vi "ABB Test Heat run.vi"(10 "Measure":enum16{"Full Load", "Partial Load", "No Load"}(ring), 11 "Heat run Type":enum16{"Full Load", "Partial- & No-Load"}(ring)) -> ()   [LabVIEW 2017]
uses:
  Temp error msg.ctl
  Video Display Buttons.ctl
  <vilib>/Analysis/baseanly.llb/Mean (DBL).vi
  ABB global.vi
  <vilib>/Analysis/NI_AALBase.lvlib
panel:
  in  "Video Displays":T1
  in  "Temp error":T2="Error: Temperature measurement "
  out "Additional Temperatures 2":string[][](table)
  out "Bearing Run readings":string[][](table)
  in  "Rated":T3
  in  "copying":string="Copying.."
  in  "copy to bearing":bool
  in  "Averaging":i32=1 min=1 max=1000
  in  "Smooth power\n    readings":bool
  in  "Reading Category":T4(ring)=enum."Wdg Temp"
  out "Power Readings":string[][](table)
  in  "Comments":string
  in  "Start":bool
  out "Type of Run":string
  out "Additional Temperatures":string[][](table)
  in  "Stabilitymessg":string="Thermal Stability reached"
  out "Time to Next reading":dbl(slide) scale=0.0..30.0 scale format="%#.1f"
  out "Start Time":dbl
  out "Temperatures":string[][](table)
  out "Readings":string[][](table)
  out "saved Readings":dbl[][](array[numeric])
  out "Serial number":string
  out "W.O number":string
  out "Norma 5000 Error":string
  in  "Record":bool
  out "Readings Table":string[][](table)
  in  "View":enum16{"Graph", "Readings"}(ring)
  out "Number readings":i32
  out "Status":enum16{"Stopped", "Running", "Finished"}(ring)
  out "Timedate":string
  in  "End test":bool
  in  "Read Mode":enum16{"Auto", "Manual"}(ring)
  in  "Exit":bool
  out "Temperature Trend":cluster{dbl[], "Best Linear Fit":dbl[]}[](graph)
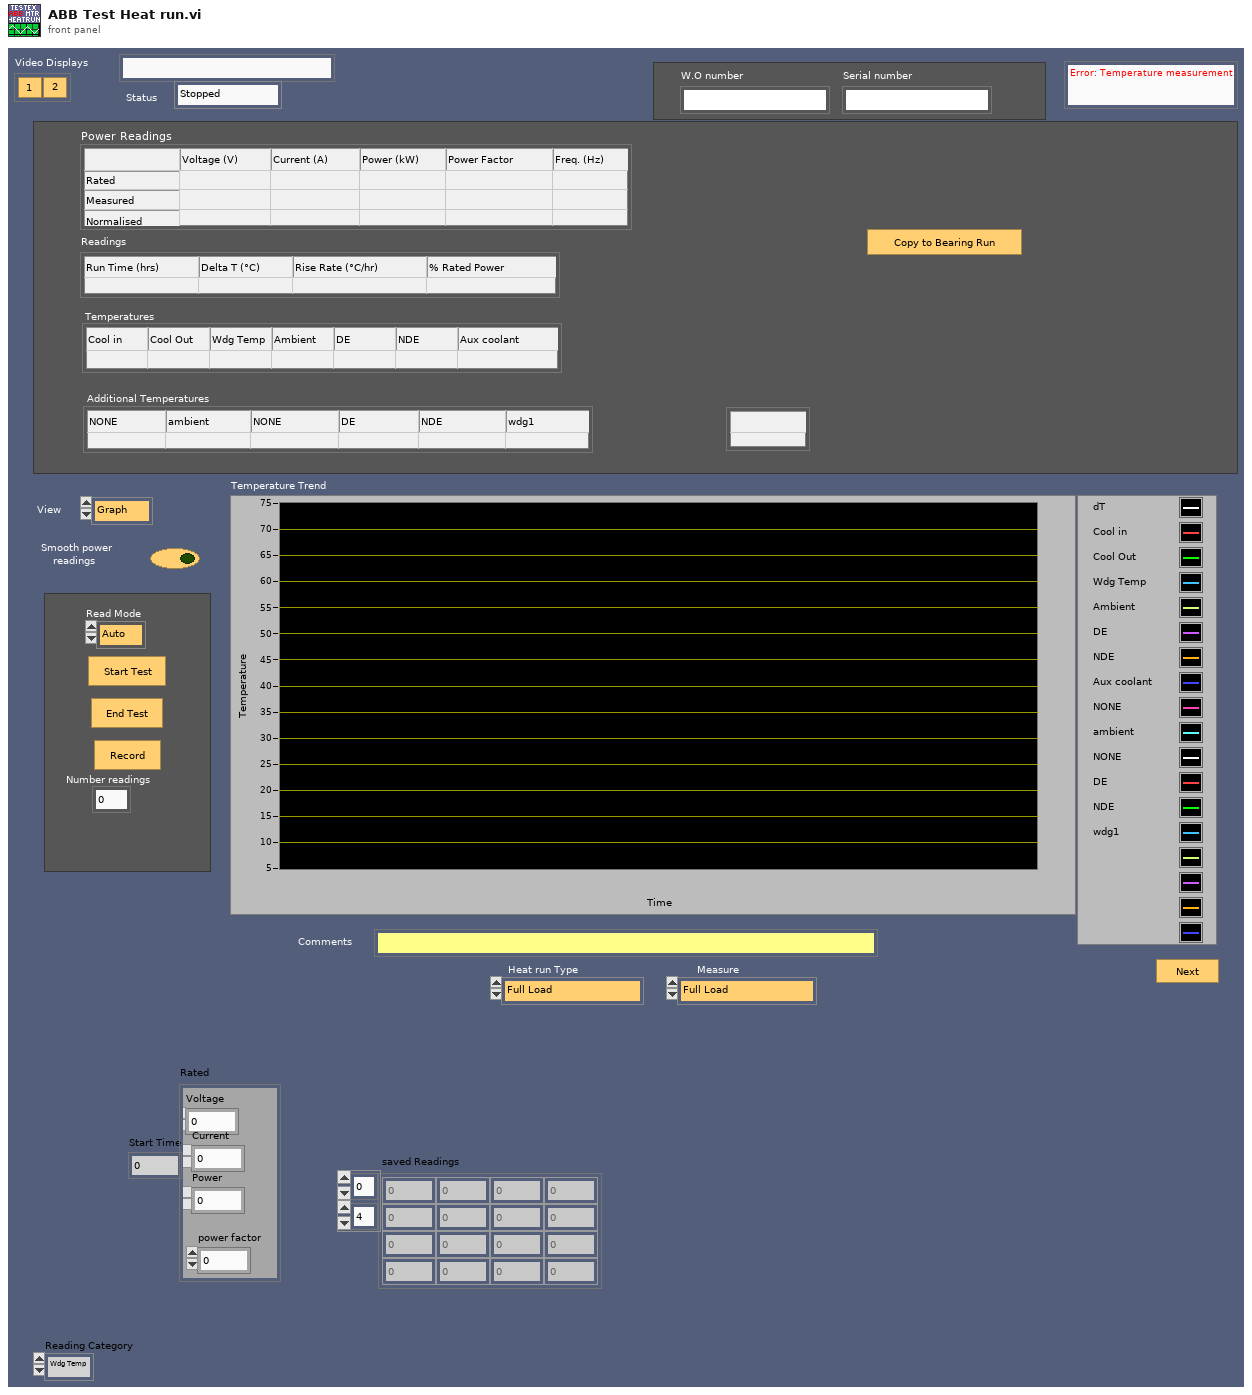
[diagram p1: front panel]
types:
  T1 = typedef "Video Display Buttons.ctl" = cluster{"1":bool, "1 2":bool}
  T2 = typedef "Temp error msg.ctl" = string
  T3 = cluster{"Voltage":dbl, "Current":dbl, "Power":dbl, "power factor":dbl}
  T4 = enum16{"None", "Cool in", "Cool Out", "Wdg Temp", "Ambient", "DE", "NDE", "Aux coolant"}
  T5 = enum16{"No load", "Locked Rotor", "Heat run", "NoLd heat run", "Partial heat run"}
  T6 = enum16{"Heat run", "Bearing run", "NoLd Heat Run", "Partial heat run"}
  T7 = cluster{"VT Primary":dbl, "VT Secondary":dbl, "CT  Primary":dbl, "CT Secondary":dbl, "Current Shunt":enum16{"Internal", "External"}, "Avg interval":dbl}
  T8 = cluster{"VT Primary":dbl, "VT Secondary":dbl, "CT  Primary":dbl, "CT Secondary":dbl, "Current Shunt":enum16{"Internal", "External"}, "Averaging interval (secs)":dbl}
  T9 = cluster{"Visa sesssion":refnum<visa-resource-name>, "error":errorcluster}
  T10 = cluster{"Simulate Norma":bool, "Norma 5000 Address":u8, "WebDaq IP Address":string, "Simulate cDAQ":bool}
  T11 = cluster{"Thermal Stability (deg/hr)":dbl, "Reading interval (mins)":dbl}
  T12 = cluster{"String":string, "String":string, "String":string, "String":string}
  T13 = cluster{"String":dbl, "String":dbl, "String":dbl, "String":dbl}
  T14 = cluster{"temp. alloc":i32[], "category":i32[], "Category names":string[], "Category none names":string[]}
  T15 = cluster{"V":dbl, "A":dbl, "W":dbl, "VA":dbl, "VAr":dbl, "Pf":dbl}
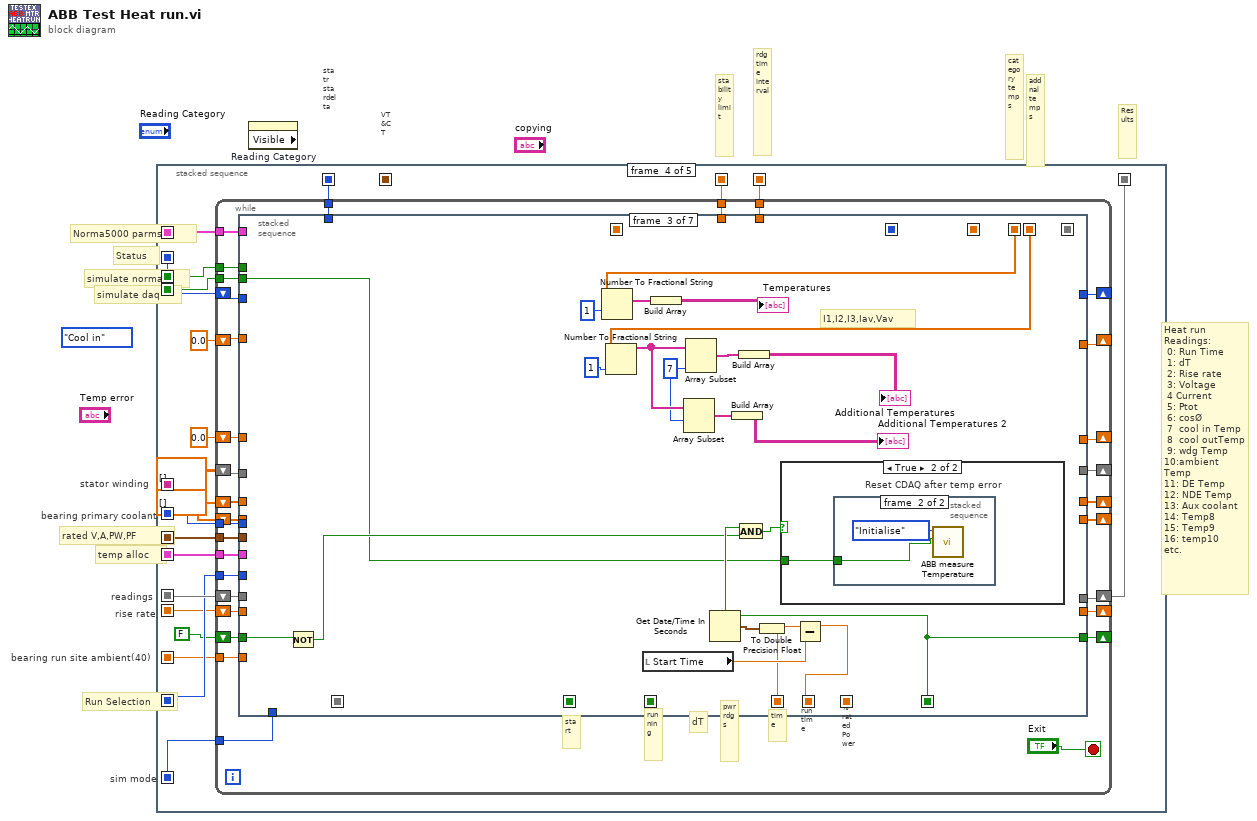
[diagram p0: block diagram]
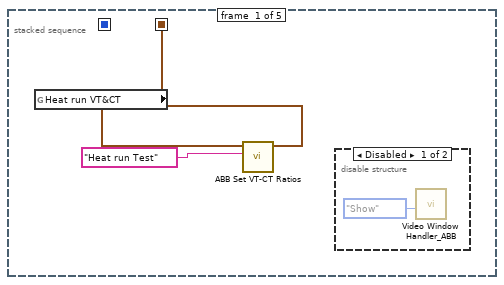
[diagram p2: hidden frame]
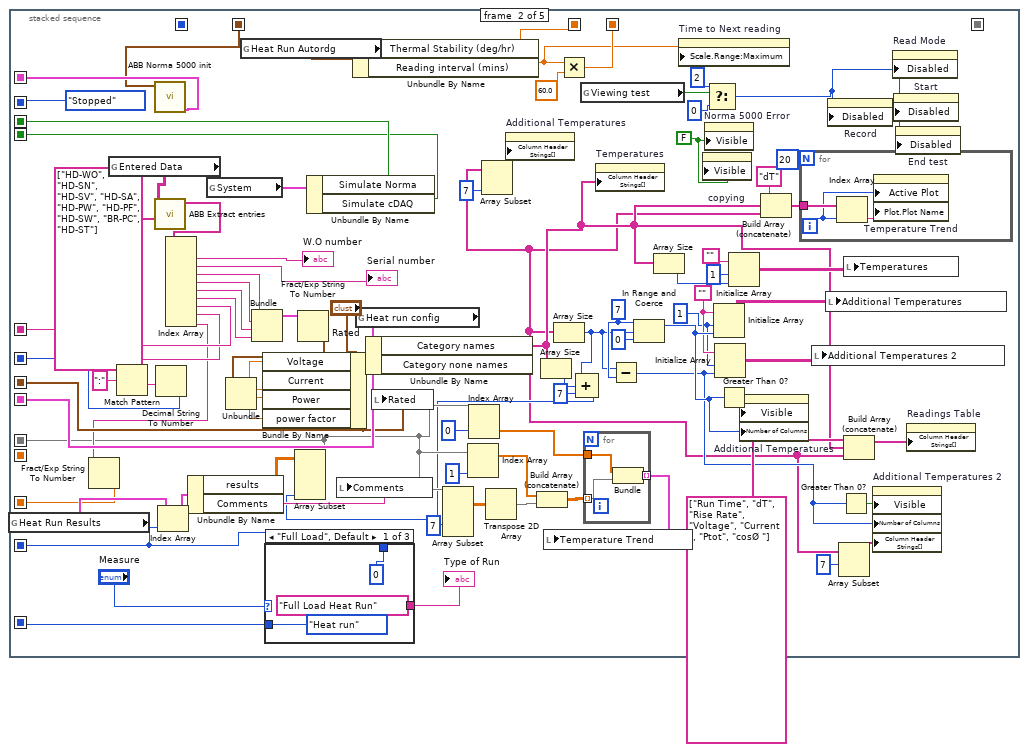
[diagram p4: hidden frame]
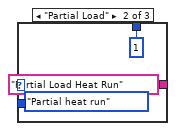
[diagram p5: hidden frame]
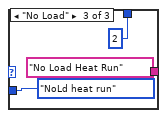
[diagram p6: hidden frame]
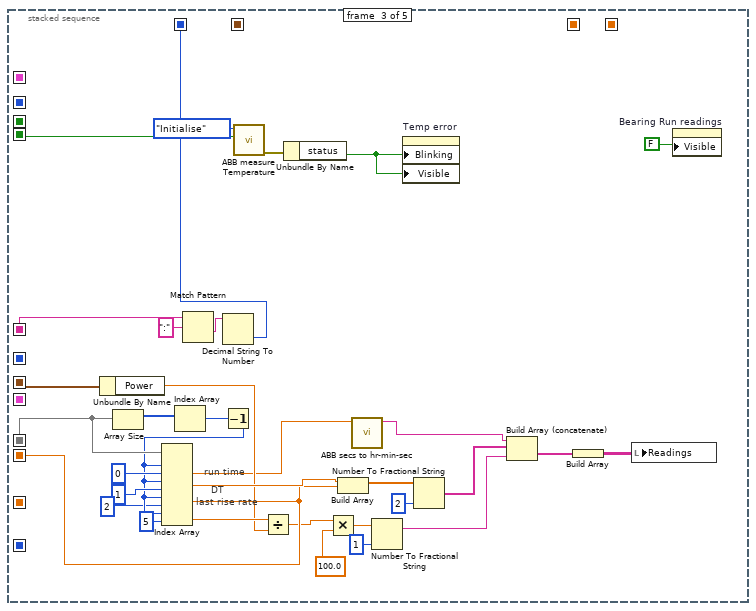
[diagram p7: hidden frame]
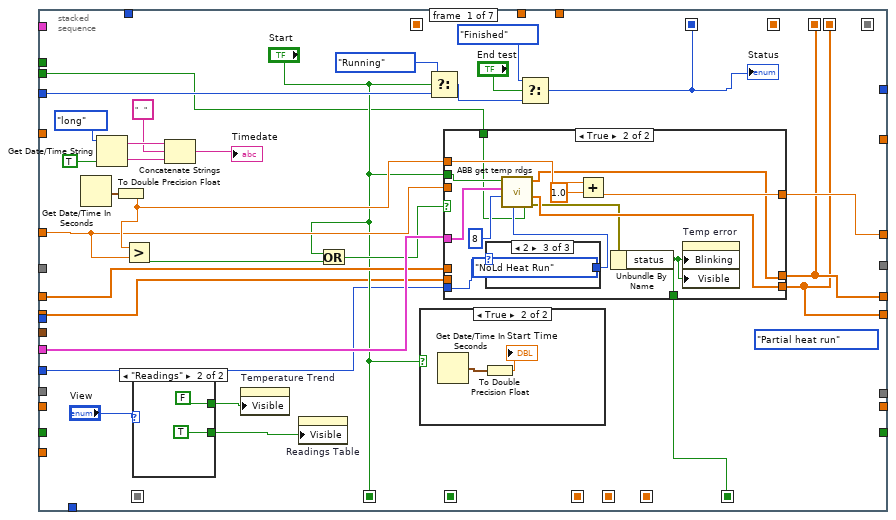
[diagram p8: hidden frame]
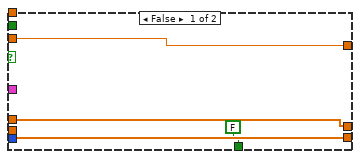
[diagram p10: hidden frame]
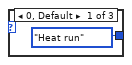
[diagram p11: hidden frame]
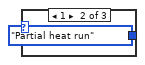
[diagram p12: hidden frame]
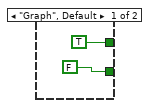
[diagram p13: hidden frame]
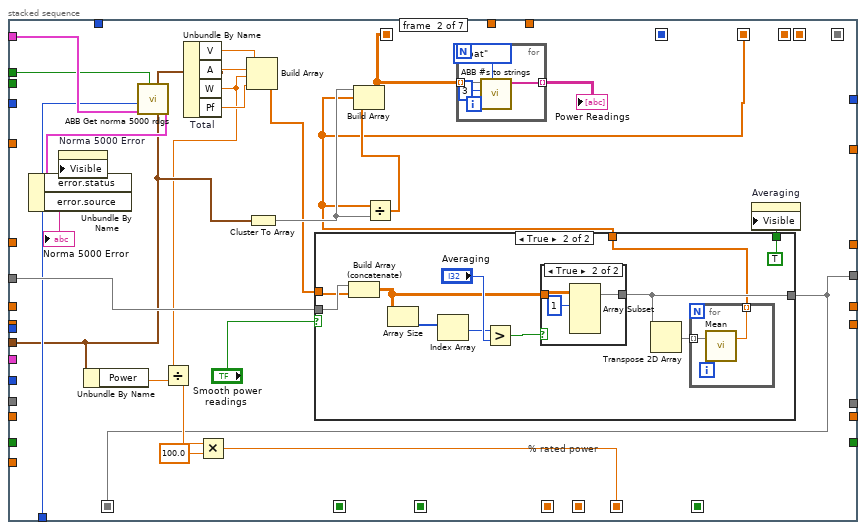
[diagram p14: hidden frame]
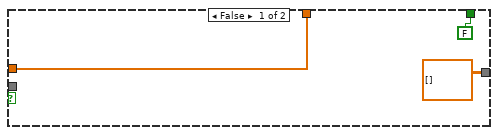
[diagram p15: hidden frame]
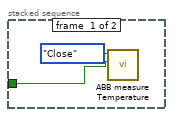
[diagram p18: hidden frame]
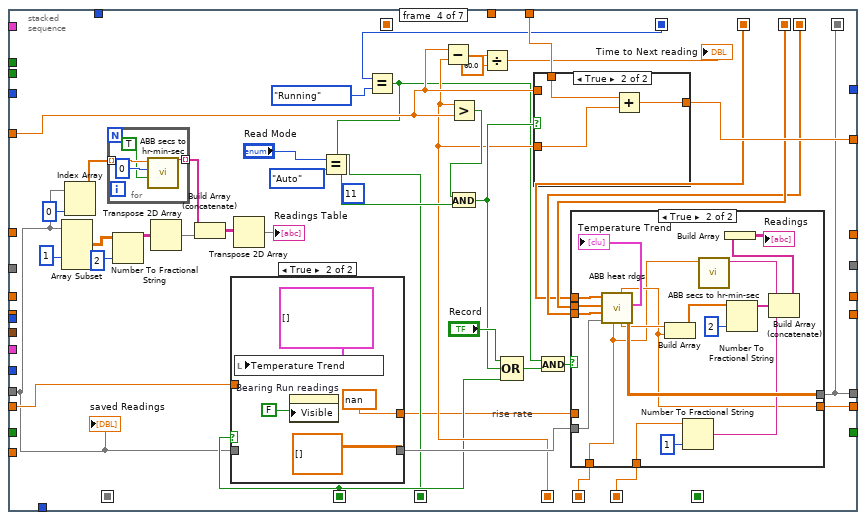
[diagram p19: hidden frame]
diagram:
  (unwired) T4."Cool in" ("Reading Category")
  # "bearing run site ambient(40)"
  # "bearing primary coolant"
  # "VT&CT"
  # "statr stardelta"
  # "stator winding"
  # "rise rate"
  # "readings"
  # "sim mode"
  # "simulate daq"
  # "addnal temps"
  # "category temps"
  # "Run Selection"
  # "stability limit"
  # "Results"
  # "rdg time interval"
  # "Heat run Readings:\n 0: Run Time\n 1: dT\n 2: Rise rate\n 3: Voltage\n 4 Current\n 5: Ptot\n 6: cosØ\n 7  cool in Temp\n 8  cool outTemp\n 9: wdg Temp\n10:ambient Temp\n11: DE Temp\n12: NDE Temp\n13: Aux coolant\n14: Temp8\n15: Temp9\n16: temp10\netc."
  # "temp alloc"
  # "rated V,A,PW,PF"
  # "simulate norma"
  # "Norma5000 parms"
  # "Status"
  n1 = stacked-sequence {
    seq-local: [_ enum16{"Stopped", "Running", "Finished"}."Stopped" ("Status") _ _ _] -> [_ _ _ w162 _]
    seq-local: [_ w91 _ _ _] -> [_ _ _ w161 w476]
    seq-local: [_ w89 _ _ _] -> [_ _ _ w160 w475]
    seq-local: [_ w39 _ _ _] -> [_ _ w130 w159 _]
    seq-local: [_ w8 _ _ _] -> [_ _ w139 w158 _]
    seq-local: [_ w54 _ _ _] -> [_ _ _ w156 _]
    seq-local: [_ w76 _ _ _] -> [_ _ _ w155 _]
    seq-local: [_ _ _ w153 _] -> [_ _ _ _ w473]
    seq-local: [_ w66 _ _ _] -> [_ _ _ w152 _]
    seq-local: [_ w48 _ _ _] -> [_ _ _ w149 w472]
    seq-local: [_ w52 _ _ _] -> [_ _ w111 w147 w469]
    seq-local: [_ w46 _ _ _] -> [_ _ _ w148 _]
    seq-local: [_ _ w133 _ _] -> [_ _ _ w146 _]
    seq-local: [_ w31 _ _ _] -> [_ _ w114 _ _]
    seq-local: [_ _ w113 _ _] -> [_ _ _ w145 _]
    seq-local: [w2 _ _ _ _] -> [_ w32 _ _ w471]
    seq-local: [_ w27 _ _ _] -> [_ _ _ w144 _]
    seq-local: [_ w25 _ _ _] -> [_ _ _ w143 _]
    frame #0 {
      n2 = global read "ABB global.vi" "Heat run VT&CT"() -> (w3:T7)
      n3 = call "ABB Set VT-CT Ratios.vi"("Test name"="Heat run Test", "VT and CT Ratios"=w3) -> ("VT and CT Ratios out"=w2:T8)  [unwired: 9 in]
      n4 = disable-structure shown="Disabled" {
        frame Disabled {
          n5 = call "Video Window Handler_ABB.vi"("Action"=enum16{"Show", "Hide", "Exit"}."Show") -> ()  [unwired: 11 in]
        }
        frame Enabled {
        }
      }
    }
    frame #1 {
      w22 = 7 ("upper limit")
      w21 = ""
      w20 = 1 ("dimension size")
      w53 = FALSE ("Visible")
      n6 = global read "ABB global.vi" "Heat Run Results"() -> (w49:cluster{"results":dbl[][], "Comments":string}[])
      n7 = global read "ABB global.vi" "Entered Data"() -> (w72:string[][])
      n8 = call "ABB Norma 5000 init.vi"("VT and CT Ratios"=w32) -> ("norma 5000 parms out"=w91:T9)  [unwired: 10 in]
      n9 = call "ABB Extract entries.vi"("Entry IDs"=string[] ["HD-WO", "HD-SN", "HD-SV", "HD-SA", "HD-PW", "HD-PF", "HD-SW", "BR-PC", "HD-ST"], "Entry table in"=w72) -> ("Selected Entries"=w38:string[])  [unwired: 9 in]
      n10 = Index Array(array=w38) -> (element #1=→"W.O number":string, element #2=→"Serial number":string, element #3=w68:string, element #4=w56:string, element #5=w55:string, element #6=w57:string, element #7=w31:string, element #8=w28:string, element #9=w26:string)  [unwired: 9 in]
      n11 = Fract/Exp String To Number(string=w26) -> (number=w25:dbl)  [unwired: 3 in, 1 out]
      n12 = Match Pattern(string=w28, regular expression=":") -> (after substring=w29:string)  [unwired: 1 in, 3 out]
      n13 = Decimal String To Number(string=w29) -> (number=w27:i32)  [unwired: 2 in, 1 out]
      n14 = global read "ABB global.vi" "System"() -> (w90:T10)
      n15 = global read "ABB global.vi" "Heat Run Autordg"() -> (w88:T11)
      n16 = Bundle("String"=w68, "String"=w56, "String"=w55, "String"=w57) -> (w67:T12)  [unwired: 1 in]
      n17 = case shown="\"Full Load\", Default" "Measure" {
        tunnel: ["Full Load Heat Run" "Partial Load Heat Run" "No Load Heat Run"] -> w51
        tunnel: [0 1 2] -> w48
        tunnel: [T5."Heat run" ("Simulate Mode") T5."Partial heat run" ("Simulate Mode") T5."NoLd heat run" ("Simulate Mode")] -> w46
        frame "Full Load", Default {
        }
        frame "Partial Load" {
        }
        frame "No Load" {
        }
      }
      "Type of Run" <- w51
      n18 = Index Array(array=w49, index=w48) -> (element=w62:cluster{"results":dbl[][], "Comments":string})
      n19 = Unbundle By Name(w62) -> ("results"=w9:dbl[][], "Comments"=w50:string)
      n20 = Fract/Exp String To Number(string=w67) -> (number=w44:T13)  [unwired: 3 in, 1 out]
      n21 = Unbundle(w44) -> ("String"=w43:dbl, "String"=w42:dbl, "String"=w41:dbl, "String"=w40:dbl)
      n22 = Bundle By Name(cluster="Rated", "Voltage"=w43, "Current"=w42, "Power"=w41, "power factor"=w40) -> (w39:T3)
      n23 = Unbundle By Name(w90) -> ("Simulate Norma"=w89:bool, "Simulate cDAQ"=w52:bool)
      n24 = local write "Comments"(w50) -> ()
      n25 = Unbundle By Name(w88) -> ("Thermal Stability (deg/hr)"=w66:dbl, "Reading interval (mins)"=w75:dbl)
      n26 = global read "ABB global.vi" "Heat run config"() -> (w54:T14)
      n27 = Unbundle By Name(w54) -> ("Category names"=w6:string[], "Category none names"=w5:string[])
      n28 = local write "Rated"(w39) -> ()
      n29 = Array Subset(array=w5, length=7) -> (w16:string[])  [unwired: 1 in]
      n30 = property on="Additional Temperatures" class="Tbl (strict)"("Column Header Strings[]"=w16) -> ()  [unwired: 2 in, 2 out]
      n31 = Array Size(array=w6) -> (size(s)=w12:i32)
      n32 = Array Size(array=w5) -> (size(s)=w11:i32)
      n33 = Multiply(x=w75, y=60.0) -> (x*y=w76:dbl)
      n34 = Compound Arithmetic op=ADD(w11, w12, 7 ("value")) -> (w7:i32)
      n35 = Array Subset(array=w9, length (col)=w7) -> (w8:dbl[][])  [unwired: 3 in]
      n36 = Array Subset(array=w8, index (col)=7 ("index")) -> (w79:dbl[][])  [unwired: 3 in]
      n37 = Index Array(array=w8, index (col)=1 ("disabled index (col)")) -> (element=w33:dbl[])  [unwired: 1 in]
      n38 = Index Array(array=w8, index (col)=0 ("disabled index (col)")) -> (element=w81:dbl[])  [unwired: 1 in]
      n39 = Transpose 2D Array(2D array=w79) -> (transposed array=w78:dbl[][])
      n40 = Build Array (concatenate)(w33, w78) -> (w34:dbl[][])
      n41 = global read "ABB global.vi" "Viewing test"() -> (w61:bool)
      n42 = for {
        tunnel: w81 -> [w104]
        tunnel: w34 -> [w103] mode=indexing
        tunnel: [w102] -> w77 mode=indexing
        n43 = Bundle(w104, w103) -> (w102:cluster{dbl[], dbl[]})  [unwired: 1 in]
      }
      n44 = local write "Temperature Trend"(w77) -> ()
      n45 = property on="Temperatures" class="Tbl (strict)"("Column Header Strings[]"=w6) -> ()  [unwired: 2 in, 2 out]
      n46 = Subtract(x=w11, y=w22) -> (x-y=w17:i32)
      n47 = In Range and Coerce(upper limit=w22, x=w11, lower limit=0) -> (coerced(x)=w24:i32)  [unwired: 1 out]
      n48 = Array Size(array=w6) -> (size(s)=w86:i32)
      n49 = property on="Time to Next reading" class="Slide (strict)"("Scale.Range:Maximum"=w75) -> ()  [unwired: 2 in, 2 out]
      n50 = property on="copying" class="Str"("Visible"=w53) -> ()  [unwired: 2 in, 2 out]
      n51 = property on="Norma 5000 Error" class="Str"("Visible"=w53) -> ()  [unwired: 2 in, 2 out]
      n52 = Select(t=2, s=w61, f=0) -> (s? t:f=w58:i32)
      n53 = Initialize Array(w21, w20, w24) -> (w65:string[][])
      n54 = Initialize Array(w21, w20, w17) -> (w19:string[][])
      n55 = Greater Than 0?(x=w24) -> (x > 0?=w64:bool)
      n56 = Initialize Array("", 1 ("dimension size"), w86) -> (w84:string[][])
      n57 = property on="Additional Temperatures" class="Tbl (strict)"("Visible"=w64, "Number of Columns"=w24) -> ()  [unwired: 2 in, 2 out]
      n58 = Build Array (concatenate)("dT", w6, w5) -> (w37:string[])
      n59 = for {
        N: 20 -> [_]
        tunnel: w37 -> [w107]
        i -> [w106]
        n60 = Index Array(array=w107, index=w106) -> (element=w105:string)
        n61 = property on="Temperature Trend" class="XYGraph (strict)"("Active Plot"=w106, "Plot.Plot Name"=w105) -> ()  [unwired: 2 in, 2 out]
      }
      n62 = local write "Additional Temperatures 2"(w19) -> ()
      n63 = local write "Additional Temperatures"(w65) -> ()
      n64 = property on="Record" class="Bool"("Disabled"=w58) -> ()  [unwired: 2 in, 2 out]
      n65 = Array Subset(array=w5, index=7) -> (w13:string[])  [unwired: 1 in]
      n66 = Greater Than 0?(x=w17) -> (x > 0?=w18:bool)
      n67 = local write "Temperatures"(w84) -> ()
      n68 = Build Array (concatenate)(string[] ["Run Time", "dT", "Rise Rate", "Voltage", "Current ", "Ptot", "cosØ "], w6, w5) -> (w73:string[])
      n69 = property on="Additional Temperatures 2" class="Tbl (strict)"("Visible"=w18, "Number of Columns"=w17, "Column Header Strings[]"=w13) -> ()  [unwired: 2 in, 2 out]
      n70 = property on="Read Mode" class="Enum (strict)"("Disabled"=w58) -> ()  [unwired: 2 in, 2 out]
      n71 = property on="Start" class="Bool"("Disabled"=w58) -> ()  [unwired: 2 in, 2 out]
      n72 = property on="End test" class="Bool"("Disabled"=w58) -> ()  [unwired: 2 in, 2 out]
      n73 = property on="Readings Table" class="Tbl (strict)"("Column Header Strings[]"=w73) -> ()  [unwired: 2 in, 2 out]
    }
    frame #2 {
      # "DT"
      # "run time"
      # "last rise rate"
      n74 = Unbundle By Name(w130) -> ("Power"=w129:dbl)
      n75 = Array Size(array=w139) -> (size(s)=w141:i32[])
      n76 = Index Array(array=w141) -> (element=w140:i32)  [unwired: 1 in]
      n77 = Match Pattern(string=w114, regular expression=":") -> (after substring=w115:string)  [unwired: 1 in, 3 out]
      n78 = Decimal String To Number(string=w115) -> (number=w113:i32)  [unwired: 2 in, 1 out]
      n79 = Decrement(x=w140) -> (x-1=w136:i32)
      n80 = Index Array(array=w139, index (row) #1=w136, index (col) #1=0, index (row) #2=w136, index (col) #2=1 ("disabled index (col)"), index (row) #3=w136, index (col) #3=2 ("disabled index (col)"), index (row) #4=w136, index (col) #4=5 ("disabled index (col)")) -> (element #1=w118:dbl, element #2=w135:dbl, element #3=w133:dbl, element #4=w131:dbl)
      n81 = call "ABB measure Temperature.vi"("Simulate"=w111, "Mode"=enum16{"Initialise", "Read", "Close"}."Initialise") -> ("error out"=w109:errorcluster)  [unwired: 7 in, 2 out]
      n82 = Divide(x=w131, y=w129) -> (x/y=w126:dbl)
      n83 = Unbundle By Name(w109) -> ("status"=w108:bool)
      n84 = Multiply(x=w126, y=100.0) -> (x*y=w120:dbl)
      n85 = Build Array(w135, w133) -> (w128:dbl[])
      n86 = call "ABB secs to hr-min-sec.vi"("Seconds"=w118) -> ("hr:min:secs"=w117:string)  [unwired: 10 in]
      n87 = Number To Fractional String(number=w120, precision (6)=i16 1) -> (F-format string=w123:string)  [unwired: 2 in]
      n88 = property on="Temp error" class="Str (strict)"("Blinking"=w108, "Visible"=w108) -> ()  [unwired: 2 in, 2 out]
      n89 = Number To Fractional String(number=w128, precision (6)=i16 2) -> (F-format string=w124:string[])  [unwired: 2 in]
      n90 = Build Array (concatenate)(w117, w124, w123) -> (w122:string[])
      n91 = Build Array(w122) -> (w121:string[][])
      n92 = local write "Readings"(w121) -> ()
      n93 = property on="Bearing Run readings" class="Tbl (strict)"("Visible"=FALSE) -> ()  [unwired: 2 in, 2 out]
    }
    frame #3 {
      w151 = dbl[] []
      n94 = while {
        shift-right: [w191] -> _
        shift-left: w162 -> [w192]
        tunnel: w161 -> [w190]
        tunnel: w160 -> [w189]
        tunnel: w159 -> [w188]
        shift-right: [w186] -> w153
        shift-left: w158 -> [w187]
        shift-right: [w183] -> _
        shift-left: 0.0 -> [w185]
        shift-right: [w184] -> _
        shift-left: w151 -> [w181]
        tunnel: w156 -> [w182]
        tunnel: w155 -> [w180]
        shift-right: [w178] -> _
        shift-left: 0.0 -> [w179]
        tunnel: w152 -> [w177]
        shift-right: [w175] -> _
        shift-left: w151 -> [w176]
        shift-right: [w173] -> _
        shift-left: dbl[][] [] -> [w174]
        tunnel: w149 -> [w172]
        tunnel: w148 -> [w171]
        tunnel: w147 -> [w170]
        shift-right: [w169] -> _
        shift-left: w146 -> [w168]
        tunnel: w145 -> [w167]
        tunnel: w144 -> [w166]
        tunnel: w143 -> [w165]
        shift-right: [w164] -> _
        shift-left: FALSE -> [w163]
        stop <- "Exit" stop-if-true
        # "run time"
        # "% rated Power"
        # "running"
        # "time"
        # "dT"
        # "pwr rdgs"
        # "start"
        n95 = stacked-sequence {
          seq-local: ["Start" _ _ _ _ _ _] -> [_ _ _ w347 _ _ _]
          seq-local: [_ w259 _ _ _ _ _] -> [_ _ _ w341 _ _ _]
          seq-local: [_ _ w317 _ _ _ _] -> [_ _ _ w352 _ _ _]
          seq-local: [w201 _ _ _ _ _ _] -> [_ _ _ w345 w403 _ _]
          seq-local: [w200 _ _ _ _ _ _] -> [_ _ w315 w344 _ _ _]
          seq-local: [_ _ _ w343 _ _ _] -> [_ _ _ _ w409 _ _]
          seq-local: [w197 _ _ _ _ _ _] -> [_ _ w313 w342 _ _ _]
          seq-local: [_ w263 _ _ _ _ _] -> [_ _ _ _ _ _ _]
          seq-local: [_ _ _ w340 _ _ _] -> [_ _ _ _ w402 w423 _]
          seq-local: [_ w251 _ _ _ _ _] -> [_ _ _ w338 _ _ _]
          seq-local: [_ w250 _ _ _ _ _] -> [_ _ _ _ _ _ _]
          seq-local: [_ _ w310 _ _ _ _] -> [_ _ _ w339 _ _ _]
          seq-local: [w194 _ _ _ _ _ _] -> [_ _ w304 _ _ _ _]
          tunnel: w192 -> [w217 _ _ _ w413 _ _]
          tunnel: [_ _ _ _ w403 _ _] -> w191
          tunnel: w190 -> [_ w275 _ _ _ _ _]
          tunnel: w189 -> [_ w271 _ _ _ _ _]
          tunnel: w188 -> [_ w256 _ _ _ _ _]
          tunnel: w187 -> [_ _ _ w333 w417 _ _]
          tunnel: [_ _ _ w340 _ _ _] -> w186
          tunnel: w185 -> [w207 _ _ _ _ _ _]
          tunnel: [w200 _ _ _ _ _ _] -> w184
          tunnel: [w206 _ _ _ _ _ _] -> w183
          tunnel: w182 -> [w205 _ _ _ _ _ _]
          tunnel: w181 -> [w204 _ _ _ _ _ _]
          tunnel: w180 -> [_ _ _ w363 _ _ _]
          tunnel: w179 -> [_ _ _ w353 _ _ _]
          tunnel: [_ _ _ w362 _ _ _] -> w178
          tunnel: w177 -> [_ _ _ _ w416 _ _]
          tunnel: w176 -> [w198 _ _ _ _ _ _]
          tunnel: [w197 _ _ _ _ _ _] -> w175
          tunnel: w174 -> [_ w262 _ _ _ _ _]
          tunnel: [_ w250 _ _ _ _ _] -> w173
          tunnel: w172 -> [w196 _ _ _ _ _ _]
          tunnel: w171 -> [_ w257 _ _ _ _ _]
          tunnel: w170 -> [w195 _ w300 _ _ _ _]
          tunnel: [_ _ _ w337 _ _ _] -> w169
          tunnel: w168 -> [_ _ _ w336 w405 _ _]
          tunnel: w167 -> [_ _ _ _ _ _ _]
          tunnel: w166 -> [_ _ _ _ _ w422 _]
          tunnel: w165 -> [_ _ _ _ _ w421 _]
          tunnel: [_ _ w304 _ _ _ _] -> w164
          tunnel: w163 -> [_ _ w303 _ _ _ _]
          frame #0 {
            (unwired) T6."Partial heat run" ("sim type")
            n96 = Get Date/Time In Seconds() -> (seconds since 1Jan1904=w209:timestamp)
            n97 = Get Date/Time String(date format (0)=enum16{"short", "long", "abbreviated"}."long", want seconds? (F)=TRUE) -> (date string=w221:string, time string=w220:string)  [unwired: 1 in]
            n98 = To Double Precision Float(number=w209) -> (double precision float=w208:dbl)
            n99 = Greater?(x=w208, y=w207) -> (0:w203:bool)
            n100 = case shown="\"Readings\"" "View" {
              tunnel: [TRUE FALSE] -> w211
              tunnel: [FALSE TRUE] -> w210
              frame "Graph", Default {
              }
              frame "Readings" {
              }
            }
            n101 = Concatenate Strings(w221, "   ", w220) -> (→"Timedate":string)
            n102 = property on="Temperature Trend" class="XYGraph (strict)"("Visible"=w211) -> ()  [unwired: 2 in, 2 out]
            n103 = property on="Readings Table" class="Tbl (strict)"("Visible"=w210) -> ()  [unwired: 2 in, 2 out]
            n104 = Or(x="Start", y=w203) -> (x .or. y?=w202:bool)
            n105 = case shown="True" "Start" {
              frame False {
              }
              frame True {
                n106 = Get Date/Time In Seconds() -> (seconds since 1Jan1904=w225:timestamp)
                n107 = To Double Precision Float(number=w225) -> (double precision float=→"Start Time":dbl)
              }
            }
            n108 = Select(t=enum16{"Stopped", "Running", "Finished"}."Running", s="Start", f=w217) -> (s? t:f=w215:enum16{"Stopped", "Running", "Finished"})
            n109 = case shown="True" w202 {
              tunnel: w208 -> [_ w242]
              tunnel: [w229 w240] -> w206
              tunnel: w207 -> [w229 _]
              tunnel: w195 -> [_ w232]
              tunnel: w205 -> [_ w238]
              tunnel: [w228 w237] -> w200
              tunnel: w204 -> [w228 _]
              tunnel: "Start" -> [_ w239]
              tunnel: w198 -> [w227 _]
              tunnel: [w227 w236] -> w197
              tunnel: w196 -> [_ w234]
              tunnel: [FALSE ("status") w230] -> w194
              frame False {
              }
              frame True {
                n110 = case shown="2" w234 {
                  tunnel: [T6."Heat run" ("sim type") T6."Partial heat run" ("sim type") T6."NoLd Heat Run" ("sim type")] -> w233
                  frame 0, Default {
                  }
                  frame 1 {
                  }
                  frame 2 {
                  }
                }
                n111 = call "ABB get temp rdgs.vi"("Sim daq"=w232, "sim type"=w233, "# categories"=8, "run config"=w238, "start"=w239) -> ("error out"=w231:errorcluster, "Category none rdgs"=w236:dbl[], "Category rdgs"=w237:dbl[])  [unwired: 3 in, 1 out]
                n112 = Add(x=w242, y=1.0) -> (x+y=w240:dbl)
                n113 = Unbundle By Name(w231) -> ("status"=w230:bool)
                n114 = property on="Temp error" class="Str (strict)"("Blinking"=w230, "Visible"=w230) -> ()  [unwired: 2 in, 2 out]
              }
            }
            n115 = Select(t=enum16{"Stopped", "Running", "Finished"}."Finished", s="End test", f=w215) -> (s? t:f=w201:enum16{"Stopped", "Running", "Finished"})
            "Status" <- w201
          }
          frame #1 {
            # "% rated power"
            n116 = Unbundle By Name(w256) -> ("Power"=w255:dbl)
            n117 = call "ABB Get norma 5000 rdgs.vi"("Rated"=w256, "simulate"=w271, "norma 5000 parms in"=w275, "Simulate Mode"=w257) -> ("norma 5000 parms out"=w272:T9, "Total"=w270:T15)  [unwired: 3 in, 3 out]
            n118 = Unbundle By Name(w272) -> ("error.status"=w274:bool, "error.source"=→"Norma 5000 Error":string)
            n119 = property on="Norma 5000 Error" class="Str"("Visible"=w274) -> ()  [unwired: 2 in, 2 out]
            n120 = Unbundle By Name "Total"(w270) -> ("V"=w266:dbl, "A"=w265:dbl, "W"=w254:dbl, "Pf"=w264:dbl)
            n121 = Divide(x=w254, y=w255) -> (x/y=w253:dbl)
            n122 = Multiply(x=w253, y=100.0) -> (x*y=w251:dbl)
            n123 = Build Array(w266, w265, w254, w264) -> (w260:dbl[])
            n124 = Cluster To Array(cluster=w256) -> (array=w267:dbl[])
            n125 = case shown="True" "Smooth power\n    readings" {
              tunnel: w262 -> [_ w283]
              tunnel: w260 -> [w278 w282]
              tunnel: [dbl[][] [] w285] -> w250
              tunnel: [w278 w284] -> w259
              tunnel: [FALSE TRUE] -> w258
              frame False {
              }
              frame True {
                n126 = Build Array (concatenate)(w283, w282) -> (w286:dbl[][])
                n127 = Array Size(array=w286) -> (size(s)=w289:i32[])
                n128 = Index Array(array=w289) -> (element=w279:i32)  [unwired: 1 in]
                n129 = Greater?(x=w279, y="Averaging") -> (0:w287:bool)
                n130 = case shown="True" w287 {
                  tunnel: w286 -> [w292 w295]
                  tunnel: [w292 w294] -> w285
                  frame False {
                  }
                  frame True {
                    n131 = Array Subset(array=w295, index (row)=1 ("index")) -> (w294:dbl[][])  [unwired: 3 in]
                  }
                }
                n132 = Transpose 2D Array(2D array=w285) -> (transposed array=w281:dbl[][])
                n133 = for {
                  tunnel: w281 -> [w291] mode=indexing
                  tunnel: [w290] -> w284 mode=indexing
                  n134 = call-poly <vilib>:"Mean.vi"("X"=w291) -> ("mean"=w290:dbl)  [unwired: 1 out]
                }
              }
            }
            n135 = Divide(x=w259, y=w267) -> (x/y=w268:dbl[])
            n136 = Build Array(w267, w259, w268) -> (w263:dbl[][])
            n137 = for {
              tunnel: w263 -> [w299] mode=indexing
              tunnel: [w296] -> w269 mode=indexing
              n138 = call "ABB #s to strings.vi"("# type"=enum16{"Float", "Relative time HH:MM"}."Float", "Precision"=3, "Numbers in"=w299) -> ("Strings out"=w296:string[])  [unwired: 8 in]
            }
            "Power Readings" <- w269
            n139 = property on="Averaging" class="DigNum (strict)"("Visible"=w258) -> ()  [unwired: 2 in, 2 out]
          }
          frame #2 {
            w305 = 7 ("length")
            # "I1,I2,I3,Iav,Vav"
            n140 = Not(x=w303) -> (.not. x?=w301:bool)
            n141 = Number To Fractional String(number=w315, precision (6)=i16 1) -> (F-format string=w314:string[])  [unwired: 2 in]
            n142 = Number To Fractional String(number=w313, precision (6)=i16 1) -> (F-format string=w308:string[])  [unwired: 2 in]
            n143 = local read "Start Time"() -> (w318:dbl)
            n144 = Build Array(w314) -> (→"Temperatures":string[][])
            n145 = Array Subset(array=w308, index=w305) -> (w306:string[])  [unwired: 1 in]
            n146 = Array Subset(array=w308, length=w305) -> (w309:string[])  [unwired: 1 in]
            n147 = Get Date/Time In Seconds() -> (seconds since 1Jan1904=w319:timestamp)
            n148 = Build Array(w306) -> (→"Additional Temperatures 2":string[][])
            n149 = And(x=w304, y=w301) -> (x .and. y?=w302:bool)
            n150 = Build Array(w309) -> (→"Additional Temperatures":string[][])
            n151 = To Double Precision Float(number=w319) -> (double precision float=w317:dbl)
            n152 = case shown="True" w302 {
              tunnel: w300 -> [_ w321]
              frame False {
              }
              frame True {
                # "Reset CDAQ after temp error"
                n153 = stacked-sequence {
                  tunnel: w321 -> [w322 w324]
                  frame #0 {
                    n154 = call "ABB measure Temperature.vi"("Simulate"=w322, "Mode"=enum16{"Initialise", "Read", "Close"}."Close") -> ()  [unwired: 7 in, 3 out]
                  }
                  frame #1 {
                    n155 = call "ABB measure Temperature.vi"("Simulate"=w324, "Mode"=enum16{"Initialise", "Read", "Close"}."Initialise") -> ()  [unwired: 7 in, 3 out]
                  }
                }
              }
            }
            n156 = Subtract(x=w317, y=w318) -> (x-y=w310:dbl)
          }
          frame #3 {
            (unwired) 11 ("index")
            # "rise rate"
            n157 = Array Subset(array=w333, index (col)=1 ("index")) -> (w334:dbl[][])  [unwired: 3 in]
            n158 = Index Array(array=w333, index (col)=0 ("disabled index (col)")) -> (element=w332:dbl[])  [unwired: 1 in]
            n159 = for {
              tunnel: w332 -> [w369] mode=indexing
              tunnel: [w367] -> w328 mode=indexing
              n160 = call "ABB secs to hr-min-sec.vi"("round off secs"=TRUE, "Precision"=i16 0, "Seconds"=w369) -> ("hr:min:secs"=w367:string)  [unwired: 8 in]
            }
            n161 = Number To Fractional String(number=w334, precision (6)=i16 2) -> (F-format string=w348:string[][])  [unwired: 2 in]
            n162 = Transpose 2D Array(2D array=w348) -> (transposed array=w327:string[][])
            n163 = Build Array (concatenate)(w328, w327) -> (w331:string[][])
            n164 = case shown="True" w347 {
              tunnel: w333 -> [w375 _]
              tunnel: [w375 dbl[][] []] -> w356
              tunnel: w336 -> [w374 _]
              tunnel: [w374 nan] -> w335
              frame False {
              }
              frame True {
                n165 = local write "Temperature Trend"(cluster{dbl[], "Best Linear Fit":dbl[]}[] [] ("Temperature Trend")) -> ()
                n166 = property on="Bearing Run readings" class="Tbl (strict)"("Visible"=FALSE) -> ()  [unwired: 2 in, 2 out]
              }
            }
            n167 = Transpose 2D Array(2D array=w331) -> (transposed array=→"Readings Table":string[][])
            n168 = Equal?(x="Read Mode", y=enum16{"Auto", "Manual"}."Auto") -> (x = y?=w359:bool)
            n169 = Equal?(x=w345, y=enum16{"Stopped", "Running", "Finished"}."Running" ("x")) -> (x = y?=w343:bool)
            n170 = Subtract(x=w353, y=w352) -> (x-y=w351:dbl)
            n171 = Greater?(x=w352, y=w353) -> (0:w358:bool)
            n172 = And(x=w358, y=w359) -> (x .and. y?=w357:bool)
            n173 = Divide(x=w351, y=60.0) -> (x/y=→"Time to Next reading":dbl)
            n174 = Compound Arithmetic op=OR("Record", w357, w347) -> (w354:bool)
            n175 = case shown="True" w357 {
              tunnel: w363 -> [_ w372]
              tunnel: w352 -> [_ w373]
              tunnel: [w370 w371] -> w362
              tunnel: w353 -> [w370 _]
              frame False {
              }
              frame True {
                n176 = Add(x=w372, y=w373) -> (x+y=w371:dbl)
              }
            }
            n177 = And(x=w343, y=w354) -> (x .and. y?=w355:bool)
            n178 = case shown="True" w355 {
              tunnel: w356 -> [w381 w396]
              tunnel: [w381 w395] -> w340
              tunnel: w341 -> [_ w399]
              tunnel: w344 -> [_ w398]
              tunnel: w342 -> [_ w394]
              tunnel: w339 -> [_ w382]
              tunnel: w338 -> [_ w383]
              tunnel: [w380 w384] -> w337
              tunnel: w335 -> [w380 _]
              frame False {
              }
              frame True {
                n179 = call "ABB heat rdgs.vi"("Run Time"=w382, "Readings in"=w396, "Addnl temps"=w394, "temperatures"=w398, "power"=w399) -> ("Readings out"=w395:dbl[][], "Temperature trend"=→"Temperature Trend":cluster{dbl[], dbl[]}[], "dT"=w387:dbl, "rise rate"=w384:dbl)  [unwired: 3 in]
                n180 = Build Array(w387, w384) -> (w391:dbl[])
                n181 = Number To Fractional String(number=w383, precision (6)=i16 1) -> (F-format string=w385:string)  [unwired: 2 in]
                n182 = call "ABB secs to hr-min-sec.vi"("Seconds"=w382) -> ("hr:min:secs"=w389:string)  [unwired: 10 in]
                n183 = Number To Fractional String(number=w391, precision (6)=i16 2) -> (F-format string=w393:string[])  [unwired: 2 in]
                n184 = Build Array (concatenate)(w389, w393, w385) -> (w392:string[])
                n185 = Build Array(w392) -> (→"Readings":string[][])
              }
            }
            "saved Readings" <- w333
          }
          frame #4 {
            n186 = Array Size(array=w417) -> (size(s)=w420:i32[])
            n187 = Index Array(array=w420) -> (element=w419:i32)  [unwired: 1 in]
            n188 = Not Equal?(x=w413, y=enum16{"Stopped", "Running", "Finished"}."Stopped") -> (x != y?=w411:bool)
            n189 = Greater?(x=w419, y=2) -> (0:w414:bool)
            n190 = Absolute Value(x=w405) -> (abs(x)=w404:dbl)
            n191 = Less?(x=w404, y=w416) -> (x < y?=w415:bool)
            n192 = Wait Until Next ms Multiple(millisecond multiple=u32 200) -> ()  [unwired: 1 out]
            n193 = Compound Arithmetic op=AND(w415, w411, w414) -> (w408:bool)
            n194 = And(x=w408, y=w409) -> (x .and. y?=w407:bool)
            n195 = Select(t=enum16{"Stopped", "Running", "Finished"}."Finished", s=w407, f=w403) -> ()  [unwired: 1 out]
            n196 = property on="Stabilitymessg" class="Str"("Visible"=w408, "Blinking"=w408) -> ()  [unwired: 2 in, 2 out]
            n197 = property on="Time to Next reading" class="Slide (strict)"("Visible"=w409) -> ()  [unwired: 2 in, 2 out]
            n198 = Array Size(array=w402) -> (size(s)=w401:i32[])
            n199 = Index Array(array=w401) -> (element=→"Number readings":i32)  [unwired: 1 in]
          }
          frame #5 {
            n200 = case shown="True" "copy to bearing" {
              tunnel: w423 -> [_ w427]
              tunnel: w422 -> [_ w426]
              tunnel: w421 -> [_ w425]
              frame False {
              }
              frame True {
                n201 = stacked-sequence {
                  tunnel: w427 -> [_ w457 _]
                  tunnel: w426 -> [_ w449 _]
                  tunnel: w425 -> [_ w443 _]
                  frame #0 {
                    w428 = TRUE ("Visible")
                    n202 = property on="copying" class="Str"("Visible"=w428) -> ()  [unwired: 2 in, 2 out]
                    n203 = property on="Bearing Run readings" class="Tbl (strict)"("Visible"=w428) -> ()  [unwired: 2 in, 2 out]
                  }
                  frame #1 {
                    w431 = 2
                    (unwired) nan
                    # "Bearing run Readings:\n 0: Run Time\n 1: DE Rise\n 2: NDE Rise\n 3:DT\n4: Cool In\n5:Ambient\n6:DE Temp\n8: NDE Temp\n9: temp\netc."
                    # "Ambient"
                    # "Aux coolant"
                    # "NDE"
                    # "DE"
                    # "Run time"
                    n204 = Index Array(array=w457, index (col) #1=0 ("disabled index (col)"), index (col) #2=11 ("index (col)"), index (col) #3=12 ("index (col)"), index (col) #4=13 ("index (col)"), index (col) #5=10 ("index (col)")) -> (element #1=w451:dbl[], element #2=w446:dbl[], element #3=w445:dbl[], element #4=w448:dbl[], element #5=w447:dbl[])  [unwired: 5 in]
                    n205 = Build Array(w448, w447, w446, w445) -> (w444:dbl[][])
                    n206 = Transpose 2D Array(2D array=w444) -> (transposed array=w432:dbl[][])
                    n207 = for {
                      tunnel: w451 -> [w461] mode=indexing
                      tunnel: w447 -> [_] mode=indexing
                      tunnel: w449 -> [w466]
                      tunnel: w432 -> [w465] mode=indexing
                      tunnel: w443 -> [w464]
                      shift-right: [w463] -> w441
                      shift-left: dbl[][] [] ("Readings out") -> [w462]
                      tunnel: [w461] -> w438
                      tunnel: [w460] -> w440
                      tunnel: [w459] -> w439
                      tunnel: [w458] -> w429
                      n208 = call "ABB bearing rdgs.vi"("Run Time"=w461, "Site ambient"=w464, "Readings in"=w462, "temperatures"=w465, "Primary coolant"=w466) -> ("Readings out"=w463:dbl[][], "NDE rise"=w459:dbl, "DE rise"=w460:dbl, "rise rate"=w458:dbl)  [unwired: 2 in, 1 out]
                    }
                    n209 = Number To Fractional String(number=w440, precision (6)=w431) -> (F-format string=w436:string)  [unwired: 2 in]
                    n210 = Number To Fractional String(number=w429, precision (6)=w431) -> (F-format string=w430:string)  [unwired: 2 in]
                    n211 = Number To Fractional String(number=w439, precision (6)=w431) -> (F-format string=w435:string)  [unwired: 2 in]
                    n212 = call "ABB secs to hr-min-sec.vi"("Seconds"=w438) -> ("hr:min:secs"=w437:string)  [unwired: 10 in]
                    n213 = Wait (ms)(milliseconds to wait=u32 1000 ("millisecond timer value")) -> ()  [unwired: 1 out]
                    n214 = global write "ABB global.vi" "Bearing run results"(w441) -> ()
                    n215 = Build Array(w437, w436, w435, w430) -> (w434:string[])
                    n216 = Build Array(w434) -> (→"Bearing Run readings":string[][])
                  }
                  frame #2 {
                    n217 = property on="copying" class="Str"("Visible"=FALSE) -> ()  [unwired: 2 in, 2 out]
                  }
                }
              }
            }
          }
          frame #6 {
            n218 = call "Video Window Handler_ABB.vi"("Video Displays"="Video Displays") -> ()  [unwired: 11 in]
          }
        }
      }
    }
    frame #4 {
      n219 = global read "ABB global.vi" "Viewing test"() -> (w474:bool)
      n220 = case shown="False" w475 {
        tunnel: w476 -> [w502 _]
        frame False {
          n221 = Unbundle By Name(w502) -> ("Visa sesssion"=w501:refnum<visa-resource-name>, "error"=w500:errorcluster)
          n222 = call "LNOPA01 Error Query.vi"("error in (no error)"=w500, "VISA session"=w501) -> ("error out"=w503:errorcluster, "dup VISA session"=w504:refnum<visa-resource-name>)  [unwired: 6 in, 2 out]
          n223 = call "LNOPA01 Close.vi"("error in (no error)"=w503, "VISA session"=w504) -> ("error out"=w505:errorcluster)  [unwired: 9 in]
          n224 = call <vilib>:"Simple Error Handler.vi"("error in (no error)"=w505) -> ()  [unwired: 4 in, 5 out]
        }
        frame True {
        }
      }
      n225 = call "ABB measure Temperature.vi"("Simulate"=w469, "Mode"=enum16{"Initialise", "Read", "Close"}."Close") -> ()  [unwired: 7 in, 3 out]
      n226 = case shown="False" w474 {
        tunnel: w473 -> [w482 _]
        tunnel: w472 -> [w480 _]
        tunnel: w471 -> [w477 _]
        frame False {
          n227 = global read "ABB global.vi" "Current test"() -> (w481:path)
          n228 = Two Button Dialog(message="Save results?", 1:"Discard" ("F button name (\"Cancel\")"), 2:"Save" ("T button name (\"OK\")")) -> (T button?=w483:bool)
          n229 = case shown="True" w483 {
            tunnel: w482 -> [_ w488]
            tunnel: w481 -> [_ w487]
            tunnel: w480 -> [_ w486]
            tunnel: w477 -> [_ w485]
            frame False {
            }
            frame True {
              n230 = stacked-sequence {
                tunnel: w488 -> [w495 _]
                tunnel: w487 -> [_ w498]
                tunnel: w486 -> [w492 _]
                tunnel: w485 -> [w489 _]
                frame #0 {
                  n231 = global write "ABB global.vi" "Heat run VT&CT"(w489) -> ()
                  n232 = global read "ABB global.vi" "Heat Run Results"() -> (w491:cluster{"results":dbl[][], "Comments":string}[])
                  n233 = global write "ABB global.vi" "Heat run Type"("Heat run Type") -> ()
                  n234 = Index Array(array=w491, index=w492) -> (element=w494:cluster{"results":dbl[][], "Comments":string})
                  n235 = Bundle By Name(cluster=w494, "results"=w495, "Comments"="Comments") -> (w497:cluster{"results":dbl[][], "Comments":string})
                  n236 = Replace Array Subset(array=w491, new element=w497, index=w492) -> (w493:cluster{"results":dbl[][], "Comments":string}[])
                  n237 = global write "ABB global.vi" "Heat Run Results"(w493) -> ()
                }
                frame #1 {
                  n238 = call "ABB Load-Save results.vi"("Path"=w498, "Mode"=enum16{"LOAD", "Save"}."Save") -> ()  [unwired: 10 in]
                }
              }
            }
          }
        }
        frame True {
        }
      }
    }
  }
  n239 = property on="Reading Category" class="Enum (strict)" props=["Visible"]() -> ()  [unwired: 2 in, 3 out]
